vi "Select ch str (SubVI).vi"(10 "字符串":string, 11 "config":T1={"initialize"=enum."SR830", "6221"={"6221 Resource"="GPIB0::24::INSTR", "Delta status"=FALSE, "电流|RMS(A)"=0.0}, "SR830+6221"={"source"=0, "Current(A)"=0.0, "阻抗(Ohm)"=0.0, "SR830 1"=FALSE, "SR830 2"=FALSE, "SR830 3"=FALSE, "SR830 4"=FALSE, "VISA 1"="", "VISA 2"="", "VISA 3"="", "VISA 4"="", "Reserve 1"=0, "Reserve 2"=-1, "Reserve 3"=-1, "Reserve 4"=-1, "Sensitivity 1"=-1, "Sensitivity 2"=0, "Sensitivity 3"=-1, "Sensitivity 4"=-1, "量程入 1"=0, "量程入 2"=0, "量程入 3"=0, "量程入 4"=0}, "2400"={"2400"=FALSE, "VISA"="", "Output Level (0)"=1e-05, "Compliance  Level (0.1)"=10.0, "ch"=[]}, "ch"={"ch"=[], "current"=[], "change?"=[], "holding current\nwhen change ch?"=FALSE, "current offset"=[]}, "Instrument"={"limit"={"Field limit"=0.0, "Field rate limit"=0.0, "Temp limit"=0.0, "Temp low limit"=0.0, "Temp rate limit "=0.0}, "genarl"={"行数"=refnum, "编辑列表框？"=refnum, "列表框"=refnum, "camg 振荡状态"=refnum, "Aborting"=refnum, "数据文件"=refnum, "warning"=refnum, "vi路径"="", "Instrument Type"=enum."PPMS-Rotate"}, "cmag"={"TM620"="TCPIP0::192.168.1.5::4266::SOCKET", "M24C Resource"="GPIB0::24::INSTR", "4G supply"="", "Temp Status 24C"=refnum, "Temp"=refnum, "9T信号"=refnum, "4g supply status"=refnum, "in-plane"="", "out-plane"="", "in-plane signal"=FALSE, "out-plane signal"=FALSE, "in plane 信号"=refnum, "pzt volt"=refnum, "camg Rate"=refnum}, "lengtou2"={"750 visa"="", "750 rotate"="", "semaphore 340"=refnum, "semaphore 750"=refnum, "750 field status"=refnum, "Input (0:A) 340"=0, "340 Resource"="GPIB0::14::INSTR", "340 Status"=refnum, "Input (0:B) 340"=1, "Loop (0: 1)"=0, "Loop (1: 1)"=0, "TCP master instance"=refnum}, "lengtou"={"TCP master instance"=refnum, "335 Status"=refnum, "335 Resource "="GPIB0::24::INSTR", "Input (0:A) 335"=0, "Input (0:B) 335"=1, "Heater Output (1:1) 335"=1, "semaphore 335"=refnum}, "325 for test"={"quantum design"=refnum, "semaphore 325"=refnum, "325 Resource "="GPIB0::13::INSTR", "Input (0:A) 325"=0, "Heater Output (1:1) 325"=1, "325 Status"=refnum}}, "2614B"={"2614B chA"=FALSE, "2614B chB"=FALSE, "VISA"=""}, "33522b"={"33522b resource name"="", "零电压"=0.0, "最大电压"=148.0, "间隔"=4.0, "最小电压"=-48.0, "loop"=0.0, "压电陶瓷电压(Vpp)"=0.0}, "gating type"=enum."2614(daul)", "层数"=0, "行数"=0, "是否处理"=[], "current 2"=[]} {"Instrument"."325 for test"."Heater Output (1:1) 325" items=["1"=1, "2"=2]; "Instrument"."325 for test"."Input (0:A) 325" items=["A", "B"]; "Instrument"."lengtou"."Heater Output (1:1) 335" items=["1"=1, "2"=2]; "Instrument"."lengtou"."Input (0:B) 335" items=["A", "B"]; "Instrument"."lengtou"."Input (0:A) 335" items=["A", "B"]; "Instrument"."lengtou2"."Loop (1: 1)" items=["1", "2"]; "Instrument"."lengtou2"."Loop (0: 1)" items=["1", "2"]; "Instrument"."lengtou2"."Input (0:B) 340" items=["A", "B", "C", "D"]; "Instrument"."lengtou2"."Input (0:A) 340" items=["A", "B", "C", "D"]; "SR830+6221"."Sensitivity 4" items=["Auto Gain"=-1, "2 nV/fA"=0, "5 nV/fA"=1, "10 nV/fA"=2, "20 nV/fA"=3, "50 nV/fA"=4, "100 nV/fA"=5, "200 nV/fA"=6, "500 nV/fA"=7, "1 uV/pA"=8, "2 uV/pA"=9, "5 uV/pA"=10, "10 uV/pA"=11, "20 uV/pA"=12, "50 uV/pA"=13, "100 uV/pA"=14, "200 uV/pA"=15, "500 uV/pA"=16, "1 mV/nA"=17, "2 mV/nA"=18, "5 mV/nA"=19, "10 mV/nA"=20, "20 mV/nA"=21, "50 mV/nA"=22, "100 mV/nA"=23, "200 mV/nA"=24, "500 mV/mA"=25, "1 V/uA"=26]; "SR830+6221"."Sensitivity 3" items=["Auto Gain"=-1, "2 nV/fA"=0, "5 nV/fA"=1, "10 nV/fA"=2, "20 nV/fA"=3, "50 nV/fA"=4, "100 nV/fA"=5, "200 nV/fA"=6, "500 nV/fA"=7, "1 uV/pA"=8, "2 uV/pA"=9, "5 uV/pA"=10, "10 uV/pA"=11, "20 uV/pA"=12, "50 uV/pA"=13, "100 uV/pA"=14, "200 uV/pA"=15, "500 uV/pA"=16, "1 mV/nA"=17, "2 mV/nA"=18, "5 mV/nA"=19, "10 mV/nA"=20, "20 mV/nA"=21, "50 mV/nA"=22, "100 mV/nA"=23, "200 mV/nA"=24, "500 mV/mA"=25, "1 V/uA"=26]; "SR830+6221"."Sensitivity 1" items=["Auto Gain"=-1, "2 nV/fA"=0, "5 nV/fA"=1, "10 nV/fA"=2, "20 nV/fA"=3, "50 nV/fA"=4, "100 nV/fA"=5, "200 nV/fA"=6, "500 nV/fA"=7, "1 uV/pA"=8, "2 uV/pA"=9, "5 uV/pA"=10, "10 uV/pA"=11, "20 uV/pA"=12, "50 uV/pA"=13, "100 uV/pA"=14, "200 uV/pA"=15, "500 uV/pA"=16, "1 mV/nA"=17, "2 mV/nA"=18, "5 mV/nA"=19, "10 mV/nA"=20, "20 mV/nA"=21, "50 mV/nA"=22, "100 mV/nA"=23, "200 mV/nA"=24, "500 mV/mA"=25, "1 V/uA"=26]; "SR830+6221"."Sensitivity 2" items=["Auto Gain"=-1, "2 nV/fA"=0, "5 nV/fA"=1, "10 nV/fA"=2, "20 nV/fA"=3, "50 nV/fA"=4, "100 nV/fA"=5, "200 nV/fA"=6, "500 nV/fA"=7, "1 uV/pA"=8, "2 uV/pA"=9, "5 uV/pA"=10, "10 uV/pA"=11, "20 uV/pA"=12, "50 uV/pA"=13, "100 uV/pA"=14, "200 uV/pA"=15, "500 uV/pA"=16, "1 mV/nA"=17, "2 mV/nA"=18, "5 mV/nA"=19, "10 mV/nA"=20, "20 mV/nA"=21, "50 mV/nA"=22, "100 mV/nA"=23, "200 mV/nA"=24, "500 mV/mA"=25, "1 V/uA"=26]; "SR830+6221"."Reserve 4" items=["Auto Gain"=-1, "2 nV/fA"=0, "5 nV/fA"=1, "10 nV/fA"=2, "20 nV/fA"=3, "50 nV/fA"=4, "100 nV/fA"=5, "200 nV/fA"=6, "500 nV/fA"=7, "1 uV/pA"=8, "2 uV/pA"=9, "5 uV/pA"=10, "10 uV/pA"=11, "20 uV/pA"=12, "50 uV/pA"=13, "100 uV/pA"=14, "200 uV/pA"=15, "500 uV/pA"=16, "1 mV/nA"=17, "2 mV/nA"=18, "5 mV/nA"=19, "10 mV/nA"=20, "20 mV/nA"=21, "50 mV/nA"=22, "100 mV/nA"=23, "200 mV/nA"=24, "500 mV/mA"=25, "1 V/uA"=26]; "SR830+6221"."Reserve 3" items=["Auto Reserve"=-1, "High Reserve"=0, "Normal"=1, "Low Noise"=2]; "SR830+6221"."Reserve 2" items=["Auto Reserve"=-1, "High Reserve"=0, "Normal"=1, "Low Noise"=2]; "SR830+6221"."Reserve 1" items=["Auto Reserve"=-1, "High Reserve"=0, "Normal"=1, "Low Noise"=2]; "SR830+6221"."source" items=["SR830 1", "SR830 2", "SR830 3", "SR830 4"]}) -> (3 "config out":T1={"initialize"=enum."SR830", "6221"={"6221 Resource"="GPIB0::24::INSTR", "Delta status"=FALSE, "电流|RMS(A)"=0.0}, "SR830+6221"={"source"=0, "Current(A)"=0.0, "阻抗(Ohm)"=0.0, "SR830 1"=FALSE, "SR830 2"=FALSE, "SR830 3"=FALSE, "SR830 4"=FALSE, "VISA 1"="", "VISA 2"="", "VISA 3"="", "VISA 4"="", "Reserve 1"=0, "Reserve 2"=-1, "Reserve 3"=-1, "Reserve 4"=-1, "Sensitivity 1"=-1, "Sensitivity 2"=0, "Sensitivity 3"=-1, "Sensitivity 4"=-1, "量程入 1"=0, "量程入 2"=0, "量程入 3"=0, "量程入 4"=0}, "2400"={"2400"=FALSE, "VISA"="", "Output Level (0)"=1e-05, "Compliance  Level (0.1)"=10.0, "ch"=[]}, "ch"={"ch"=[], "current"=[], "change?"=[], "holding current\nwhen change ch?"=FALSE, "current offset"=[]}, "Instrument"={"limit"={"Field limit"=0.0, "Field rate limit"=0.0, "Temp limit"=0.0, "Temp low limit"=0.0, "Temp rate limit "=0.0}, "genarl"={"行数"=refnum, "编辑列表框？"=refnum, "列表框"=refnum, "camg 振荡状态"=refnum, "Aborting"=refnum, "数据文件"=refnum, "warning"=refnum, "vi路径"="", "Instrument Type"=enum."PPMS-Rotate"}, "cmag"={"TM620"="TCPIP0::192.168.1.5::4266::SOCKET", "M24C Resource"="GPIB0::24::INSTR", "4G supply"="", "Temp Status 24C"=refnum, "Temp"=refnum, "9T信号"=refnum, "4g supply status"=refnum, "in-plane"="", "out-plane"="", "in-plane signal"=FALSE, "out-plane signal"=FALSE, "in plane 信号"=refnum, "pzt volt"=refnum, "camg Rate"=refnum}, "lengtou2"={"750 visa"="", "750 rotate"="", "semaphore 340"=refnum, "semaphore 750"=refnum, "750 field status"=refnum, "Input (0:A) 340"=0, "340 Resource"="GPIB0::14::INSTR", "340 Status"=refnum, "Input (0:B) 340"=1, "Loop (0: 1)"=0, "Loop (1: 1)"=0, "TCP master instance"=refnum}, "lengtou"={"TCP master instance"=refnum, "335 Status"=refnum, "335 Resource "="GPIB0::24::INSTR", "Input (0:A) 335"=0, "Input (0:B) 335"=1, "Heater Output (1:1) 335"=1, "semaphore 335"=refnum}, "325 for test"={"quantum design"=refnum, "semaphore 325"=refnum, "325 Resource "="GPIB0::13::INSTR", "Input (0:A) 325"=0, "Heater Output (1:1) 325"=1, "325 Status"=refnum}}, "2614B"={"2614B chA"=FALSE, "2614B chB"=FALSE, "VISA"=""}, "33522b"={"33522b resource name"="", "零电压"=0.0, "最大电压"=148.0, "间隔"=4.0, "最小电压"=-48.0, "loop"=0.0, "压电陶瓷电压(Vpp)"=0.0}, "gating type"=enum."2614(daul)", "层数"=0, "行数"=0, "是否处理"=[], "current 2"=[]} {"Instrument"."325 for test"."Heater Output (1:1) 325" items=["1"=1, "2"=2]; "Instrument"."325 for test"."Input (0:A) 325" items=["A", "B"]; "Instrument"."lengtou"."Heater Output (1:1) 335" items=["1"=1, "2"=2]; "Instrument"."lengtou"."Input (0:B) 335" items=["A", "B"]; "Instrument"."lengtou"."Input (0:A) 335" items=["A", "B"]; "Instrument"."lengtou2"."Loop (1: 1)" items=["1", "2"]; "Instrument"."lengtou2"."Loop (0: 1)" items=["1", "2"]; "Instrument"."lengtou2"."Input (0:B) 340" items=["A", "B", "C", "D"]; "Instrument"."lengtou2"."Input (0:A) 340" items=["A", "B", "C", "D"]; "SR830+6221"."Sensitivity 4" items=["Auto Gain"=-1, "2 nV/fA"=0, "5 nV/fA"=1, "10 nV/fA"=2, "20 nV/fA"=3, "50 nV/fA"=4, "100 nV/fA"=5, "200 nV/fA"=6, "500 nV/fA"=7, "1 uV/pA"=8, "2 uV/pA"=9, "5 uV/pA"=10, "10 uV/pA"=11, "20 uV/pA"=12, "50 uV/pA"=13, "100 uV/pA"=14, "200 uV/pA"=15, "500 uV/pA"=16, "1 mV/nA"=17, "2 mV/nA"=18, "5 mV/nA"=19, "10 mV/nA"=20, "20 mV/nA"=21, "50 mV/nA"=22, "100 mV/nA"=23, "200 mV/nA"=24, "500 mV/mA"=25, "1 V/uA"=26]; "SR830+6221"."Sensitivity 3" items=["Auto Gain"=-1, "2 nV/fA"=0, "5 nV/fA"=1, "10 nV/fA"=2, "20 nV/fA"=3, "50 nV/fA"=4, "100 nV/fA"=5, "200 nV/fA"=6, "500 nV/fA"=7, "1 uV/pA"=8, "2 uV/pA"=9, "5 uV/pA"=10, "10 uV/pA"=11, "20 uV/pA"=12, "50 uV/pA"=13, "100 uV/pA"=14, "200 uV/pA"=15, "500 uV/pA"=16, "1 mV/nA"=17, "2 mV/nA"=18, "5 mV/nA"=19, "10 mV/nA"=20, "20 mV/nA"=21, "50 mV/nA"=22, "100 mV/nA"=23, "200 mV/nA"=24, "500 mV/mA"=25, "1 V/uA"=26]; "SR830+6221"."Sensitivity 1" items=["Auto Gain"=-1, "2 nV/fA"=0, "5 nV/fA"=1, "10 nV/fA"=2, "20 nV/fA"=3, "50 nV/fA"=4, "100 nV/fA"=5, "200 nV/fA"=6, "500 nV/fA"=7, "1 uV/pA"=8, "2 uV/pA"=9, "5 uV/pA"=10, "10 uV/pA"=11, "20 uV/pA"=12, "50 uV/pA"=13, "100 uV/pA"=14, "200 uV/pA"=15, "500 uV/pA"=16, "1 mV/nA"=17, "2 mV/nA"=18, "5 mV/nA"=19, "10 mV/nA"=20, "20 mV/nA"=21, "50 mV/nA"=22, "100 mV/nA"=23, "200 mV/nA"=24, "500 mV/mA"=25, "1 V/uA"=26]; "SR830+6221"."Sensitivity 2" items=["Auto Gain"=-1, "2 nV/fA"=0, "5 nV/fA"=1, "10 nV/fA"=2, "20 nV/fA"=3, "50 nV/fA"=4, "100 nV/fA"=5, "200 nV/fA"=6, "500 nV/fA"=7, "1 uV/pA"=8, "2 uV/pA"=9, "5 uV/pA"=10, "10 uV/pA"=11, "20 uV/pA"=12, "50 uV/pA"=13, "100 uV/pA"=14, "200 uV/pA"=15, "500 uV/pA"=16, "1 mV/nA"=17, "2 mV/nA"=18, "5 mV/nA"=19, "10 mV/nA"=20, "20 mV/nA"=21, "50 mV/nA"=22, "100 mV/nA"=23, "200 mV/nA"=24, "500 mV/mA"=25, "1 V/uA"=26]; "SR830+6221"."Reserve 4" items=["Auto Gain"=-1, "2 nV/fA"=0, "5 nV/fA"=1, "10 nV/fA"=2, "20 nV/fA"=3, "50 nV/fA"=4, "100 nV/fA"=5, "200 nV/fA"=6, "500 nV/fA"=7, "1 uV/pA"=8, "2 uV/pA"=9, "5 uV/pA"=10, "10 uV/pA"=11, "20 uV/pA"=12, "50 uV/pA"=13, "100 uV/pA"=14, "200 uV/pA"=15, "500 uV/pA"=16, "1 mV/nA"=17, "2 mV/nA"=18, "5 mV/nA"=19, "10 mV/nA"=20, "20 mV/nA"=21, "50 mV/nA"=22, "100 mV/nA"=23, "200 mV/nA"=24, "500 mV/mA"=25, "1 V/uA"=26]; "SR830+6221"."Reserve 3" items=["Auto Reserve"=-1, "High Reserve"=0, "Normal"=1, "Low Noise"=2]; "SR830+6221"."Reserve 2" items=["Auto Reserve"=-1, "High Reserve"=0, "Normal"=1, "Low Noise"=2]; "SR830+6221"."Reserve 1" items=["Auto Reserve"=-1, "High Reserve"=0, "Normal"=1, "Low Noise"=2]; "SR830+6221"."source" items=["SR830 1", "SR830 2", "SR830 3", "SR830 4"]})   [LabVIEW 2019, in "Take Seq.lvlib"]
uses:
  Take Seq.lvlib
  ctl/config.ctl
  <vilib>/NI/Modbus Library/API/Master/Modbus Master.lvclass
  ctl/initialize.ctl
  ctl/Instrument.ctl
  ctl/limit.ctl
  ctl/warning.ctl
  ctl/Instrument Type.ctl
  ctl/335 state.ctl
  ctl/9T mag field stauts.ctl
  C:/Users/fuyang/Desktop/postdoctor/labview/labview-measure/lib/QDInstrument.dll
  lib/QDInstrument.dll
  ctl/Gating type.ctl
  SubVI.lvlib
  lib/Keithley 622x/Keithley 622x.lvlib
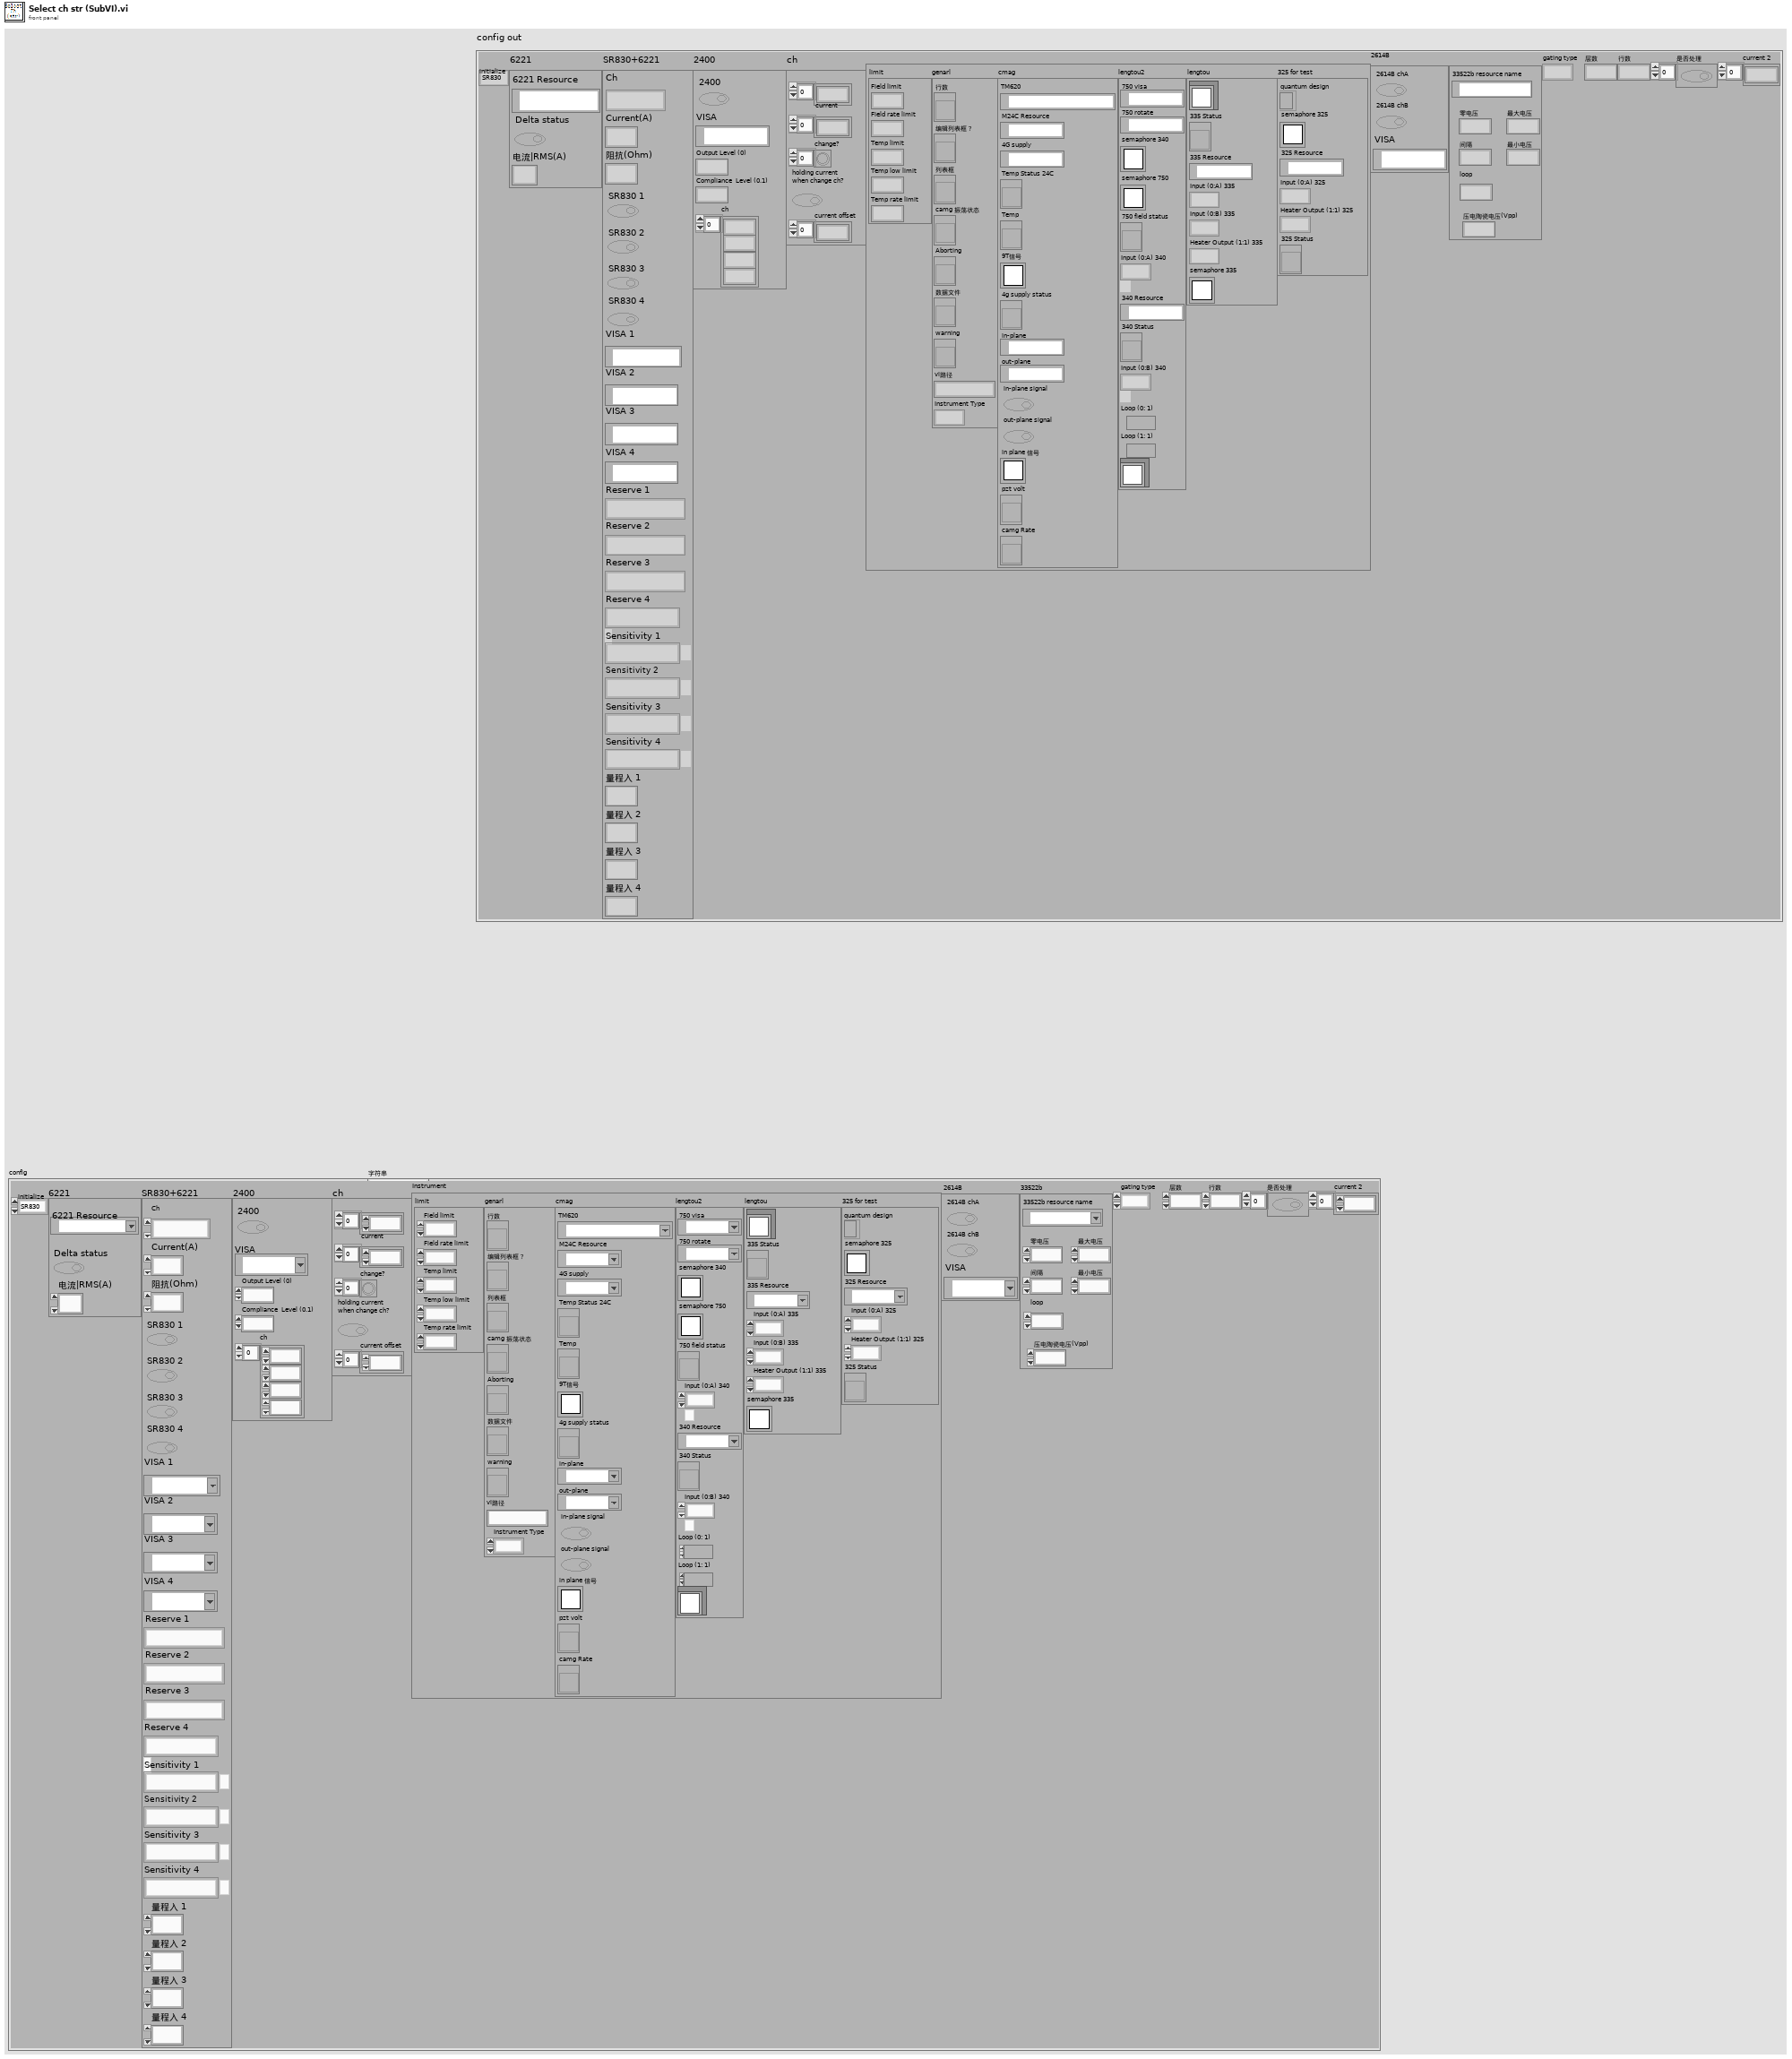
[diagram p1: front panel]
types:
  T1 = typedef "config.ctl" = cluster{"initialize":T2, "6221":cluster{"6221 Resource":refnum<visa-resource-name>, "Delta status":bool, "电流|RMS(A)":dbl}, "SR830+6221":cluster{"source":u16, "Current(A)":dbl, "阻抗(Ohm)":dbl, "SR830 1":bool, "SR830 2":bool, "SR830 3":bool, "SR830 4":bool, "VISA 1":refnum<visa-resource-name>, "VISA 2":refnum<visa-resource-name>, "VISA 3":refnum<visa-resource-name>, "VISA 4":refnum<visa-resource-name>, "Reserve 1":i16, "Reserve 2":i16, "Reserve 3":i16, "Reserve 4":i16, "Sensitivity 1":i16, "Sensitivity 2":i16, "Sensitivity 3":i16, "Sensitivity 4":i16, "量程入 1":i32, "量程入 2":i32, "量程入 3":i32, "量程入 4":i32}, "2400":cluster{"2400":bool, "VISA":refnum<visa-resource-name>, "Output Level (0)":dbl, "Compliance  Level (0.1)":dbl, "ch":i32[]}, "ch":cluster{"ch":i32[], "current":dbl[], "change?":bool[], "holding current\nwhen change ch?":bool, "current offset":dbl[]}, "Instrument":T3, "2614B":cluster{"2614B chA":bool, "2614B chB":bool, "VISA":refnum<visa-resource-name>}, "33522b":cluster{"33522b resource name":refnum<visa-resource-name>, "零电压":dbl, "最大电压":dbl, "间隔":dbl, "最小电压":dbl, "loop":dbl, "压电陶瓷电压(Vpp)":dbl}, "gating type":T7, "层数":i32, "行数":i32, "是否处理":bool[], "current 2":dbl[]}
  T2 = typedef "initialize.ctl" = enum16{"SR830", "keithley6221-SR830", "Delta", "Delta-tunnelling", "keithley6221-2182-DC", "PZT", "4200"}
  T3 = typedef "Instrument.ctl" = cluster{"limit":T4, "genarl":cluster{"行数":refnum<vi>, "编辑列表框？":refnum<vi>, "列表框":refnum<vi>, "camg 振荡状态":refnum<vi>, "Aborting":refnum<vi>, "数据文件":refnum<vi>, "warning":refnum<vi>, "vi路径":string, "Instrument Type":T5}, "cmag":cluster{"TM620":refnum<visa-resource-name>, "M24C Resource":refnum<visa-resource-name>, "4G supply":refnum<visa-resource-name>, "Temp Status 24C":refnum<vi>, "Temp":refnum<vi>, "9T信号":T6, "4g supply status":refnum<vi>, "in-plane":refnum<visa-resource-name>, "out-plane":refnum<visa-resource-name>, "in-plane signal":bool, "out-plane signal":bool, "in plane 信号":T6, "pzt volt":refnum<vi>, "camg Rate":refnum<vi>}, "lengtou2":cluster{"750 visa":refnum<visa-resource-name>, "750 rotate":refnum<visa-resource-name>, "semaphore 340":T6, "semaphore 750":T6, "750 field status":refnum<vi>, "Input (0:A) 340":u16, "340 Resource":refnum<visa-resource-name>, "340 Status":refnum<vi>, "Input (0:B) 340":u16, "Loop (0: 1)":u16, "Loop (1: 1)":u16, "TCP master instance":refnum<class "Modbus Master.lvclass">}, "lengtou":cluster{"TCP master instance":refnum<class "Modbus Master.lvclass">, "335 Status":refnum<vi>, "335 Resource ":refnum<visa-resource-name>, "Input (0:A) 335":u16, "Input (0:B) 335":u16, "Heater Output (1:1) 335":u16, "semaphore 335":T6}, "325 for test":cluster{"quantum design":refnum<k24>, "semaphore 325":T6, "325 Resource ":refnum<visa-resource-name>, "Input (0:A) 325":u16, "Heater Output (1:1) 325":u16, "325 Status":refnum<vi>}}
  T4 = typedef "limit.ctl" = cluster{"Field limit":dbl, "Field rate limit":dbl, "Temp limit":dbl, "Temp low limit":dbl, "Temp rate limit ":dbl}
  T5 = typedef "Instrument Type.ctl" = enum16{"PPMS", "VersaLab", "DynaCool", "SVSM", "PPMS-Rotate", "Lakeshore335", "lengtou2", "9T mag old", "9T cmag", "9T cmag DAC", "9T cmag rotate", "test"}
  T6 = typedef "Semaphore RefNum" = refnum<k1>
  T7 = typedef "Gating type.ctl" = enum32{"null", "2614(daul)", "2400", "6517B"}
  T8 = cluster{"ch":i32[], "current":dbl[], "change?":bool[], "holding current\nwhen change ch?":bool, "current offset":dbl[]}
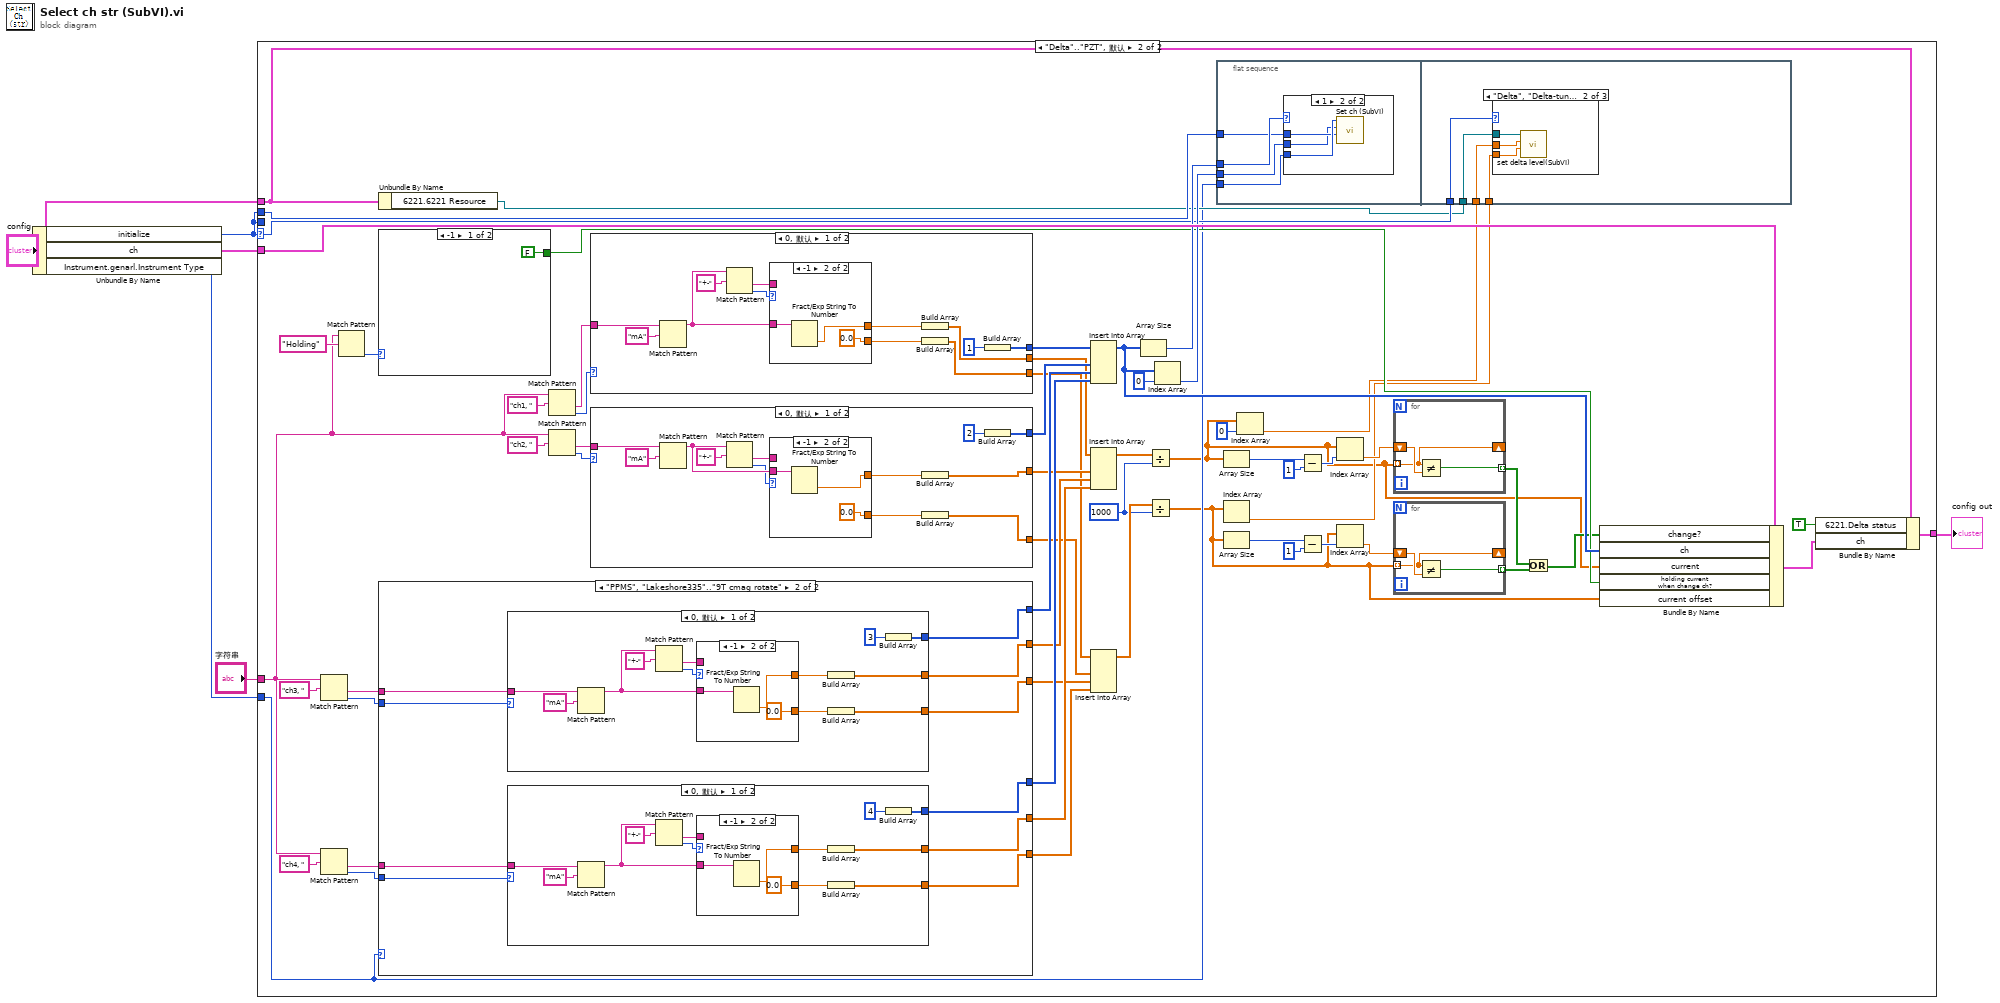
[diagram p0: block diagram]
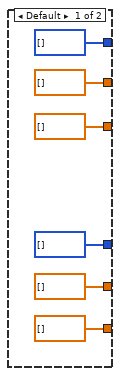
[diagram p3: hidden frame]
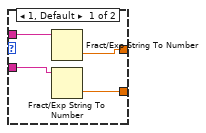
[diagram p4: hidden frame]
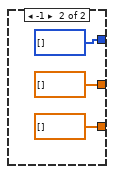
[diagram p5: hidden frame]
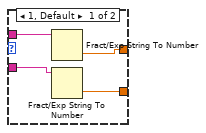
[diagram p6: hidden frame]
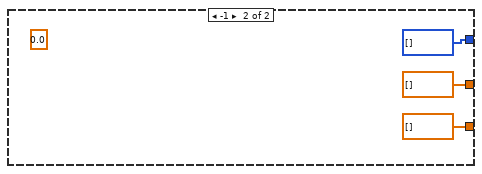
[diagram p7: hidden frame]
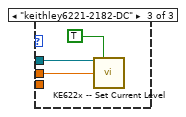
[diagram p10: hidden frame]
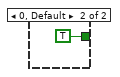
[diagram p11: hidden frame]
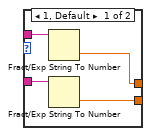
[diagram p12: hidden frame]
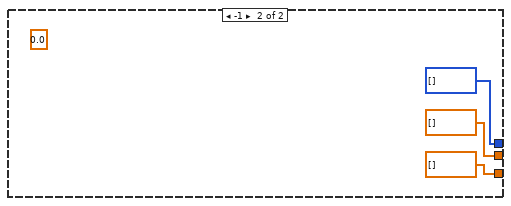
[diagram p13: hidden frame]
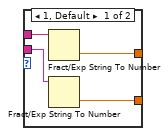
[diagram p14: hidden frame]
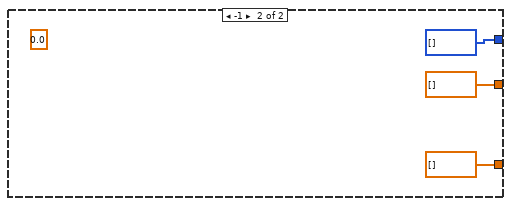
[diagram p15: hidden frame]
diagram:
  n1 = Unbundle By Name("config") -> ("initialize"=w2:T2, "ch"=w3:T8, "Instrument.genarl.Instrument Type"=w1:T5)
  n2 = case shown="\"Delta\"..\"PZT\", 默认" w2 {
    selector: w2 -> [_ w28]
    tunnel: "字符串" -> [_ w30]
    tunnel: w2 -> [_ _]
    tunnel: "config" -> [w7 w52]
    tunnel: [w7 w50] -> w4
    tunnel: w3 -> [_ w61]
    tunnel: w2 -> [_ w46]
    tunnel: w1 -> [_ w25]
    frame "SR830", "keithley6221-SR830" {
    }
    frame "Delta".."PZT", Default {
      w9 = 1000
      n3 = Match Pattern(string=w30, regular expression="ch3, " ("正则表达式")) -> (after substring=w58:string, offset past match=w55:i32)  [unwired: 1 in, 2 out]
      n4 = Match Pattern(string=w30, regular expression="ch4, " ("正则表达式")) -> (after substring=w57:string, offset past match=w56:i32)  [unwired: 1 in, 2 out]
      n5 = Match Pattern(string=w30, regular expression="Holding" ("正则表达式")) -> (offset past match=w31:i32)  [unwired: 1 in, 3 out]
      n6 = Unbundle By Name(w52) -> ("6221.6221 Resource"=w27:refnum<visa-resource-name>)
      n7 = case shown="-1" w31 {
        tunnel: [FALSE TRUE] -> w29
        frame -1 {
        }
        frame 0, Default {
        }
      }
      n8 = case shown="\"PPMS\", \"Lakeshore335\"..\"9T cmag rotate\"" w25 {
        tunnel: w58 -> [_ w86]
        tunnel: w57 -> [_ w85]
        tunnel: w56 -> [_ w84]
        tunnel: w55 -> [_ w83]
        tunnel: [i32[] [] w82] -> w42
        tunnel: [i32[] [] w81] -> w41
        tunnel: [dbl[] [] w80] -> w37
        tunnel: [dbl[] [] w79] -> w36
        tunnel: [dbl[] [] w78] -> w22
        tunnel: [dbl[] [] w77] -> w21
        frame Default {
        }
        frame "PPMS", "Lakeshore335".."9T cmag rotate" {
          n9 = case shown="0, 默认" w83 {
            tunnel: w86 -> [w120 _]
            tunnel: [w116 dbl[] []] -> w80
            tunnel: [w117 i32[] []] -> w82
            tunnel: [w114 dbl[] []] -> w78
            frame 0, Default {
              n10 = Match Pattern(string=w120, regular expression="mA" ("正则表达式")) -> (before substring=w112:string)  [unwired: 1 in, 3 out]
              n11 = Match Pattern(string=w112, regular expression="+-" ("正则表达式")) -> (after substring=w113:string, offset past match=w111:i32)  [unwired: 1 in, 2 out]
              n12 = case shown="-1" w111 {
                tunnel: w113 -> [w124 _]
                tunnel: w112 -> [w123 w127]
                tunnel: [w122 0.0] -> w109
                tunnel: [w121 w126] -> w110
                frame 1, Default {
                  n13 = Fract/Exp String To Number(string=w124) -> (number=w121:dbl)  [unwired: 3 in, 1 out]
                  n14 = Fract/Exp String To Number(string=w123) -> (number=w122:dbl)  [unwired: 3 in, 1 out]
                }
                frame -1 {
                  n15 = Fract/Exp String To Number(string=w127) -> (number=w126:dbl)  [unwired: 3 in, 1 out]
                }
              }
              n16 = Build Array(w110) -> (w116:dbl[])
              n17 = Build Array(w109) -> (w114:dbl[])
              n18 = Build Array(3) -> (w117:i32[])
            }
            frame -1 {
              (unwired) 0.0
            }
          }
          n19 = case shown="0, 默认" w84 {
            tunnel: w85 -> [w98 _]
            tunnel: [w94 dbl[] []] -> w79
            tunnel: [w95 i32[] []] -> w81
            tunnel: [w92 dbl[] []] -> w77
            frame 0, Default {
              n20 = Match Pattern(string=w98, regular expression="mA" ("正则表达式")) -> (before substring=w90:string)  [unwired: 1 in, 3 out]
              n21 = Match Pattern(string=w90, regular expression="+-" ("正则表达式")) -> (after substring=w91:string, offset past match=w87:i32)  [unwired: 1 in, 2 out]
              n22 = case shown="-1" w87 {
                tunnel: w91 -> [w102 _]
                tunnel: w90 -> [w101 w105]
                tunnel: [w100 0.0] -> w89
                tunnel: [w99 w104] -> w88
                frame 1, Default {
                  n23 = Fract/Exp String To Number(string=w102) -> (number=w99:dbl)  [unwired: 3 in, 1 out]
                  n24 = Fract/Exp String To Number(string=w101) -> (number=w100:dbl)  [unwired: 3 in, 1 out]
                }
                frame -1 {
                  n25 = Fract/Exp String To Number(string=w105) -> (number=w104:dbl)  [unwired: 3 in, 1 out]
                }
              }
              n26 = Build Array(w88) -> (w94:dbl[])
              n27 = Build Array(w89) -> (w92:dbl[])
              n28 = Build Array(4) -> (w95:i32[])
            }
            frame -1 {
            }
          }
        }
      }
      n29 = Match Pattern(string=w30, regular expression="ch1, " ("正则表达式")) -> (after substring=w59:string, offset past match=w60:i32)  [unwired: 1 in, 2 out]
      n30 = Match Pattern(string=w30, regular expression="ch2, " ("正则表达式")) -> (after substring=w62:string, offset past match=w63:i32)  [unwired: 1 in, 2 out]
      n31 = case shown="0, 默认" w60 {
        tunnel: w59 -> [w164 _]
        tunnel: [w160 dbl[] []] -> w39
        tunnel: [w161 i32[] []] -> w44
        tunnel: [w158 dbl[] []] -> w24
        frame 0, Default {
          n32 = Match Pattern(string=w164, regular expression="mA" ("正则表达式")) -> (before substring=w157:string)  [unwired: 1 in, 3 out]
          n33 = Match Pattern(string=w157, regular expression="+-" ("正则表达式")) -> (after substring=w156:string, offset past match=w153:i32)  [unwired: 1 in, 2 out]
          n34 = case shown="-1" w153 {
            tunnel: w156 -> [w168 _]
            tunnel: w157 -> [w167 w171]
            tunnel: [w166 0.0] -> w154
            tunnel: [w165 w170] -> w155
            frame 1, Default {
              n35 = Fract/Exp String To Number(string=w168) -> (number=w165:dbl)  [unwired: 3 in, 1 out]
              n36 = Fract/Exp String To Number(string=w167) -> (number=w166:dbl)  [unwired: 3 in, 1 out]
            }
            frame -1 {
              n37 = Fract/Exp String To Number(string=w171) -> (number=w170:dbl)  [unwired: 3 in, 1 out]
            }
          }
          n38 = Build Array(w155) -> (w160:dbl[])
          n39 = Build Array(w154) -> (w158:dbl[])
          n40 = Build Array(1) -> (w161:i32[])
        }
        frame -1 {
          (unwired) 0.0
        }
      }
      n41 = case shown="0, 默认" w63 {
        tunnel: w62 -> [w186 _]
        tunnel: [w182 dbl[] []] -> w38
        tunnel: [w183 i32[] []] -> w43
        tunnel: [w180 dbl[] []] -> w23
        frame 0, Default {
          n42 = Match Pattern(string=w186, regular expression="mA" ("正则表达式")) -> (before substring=w178:string)  [unwired: 1 in, 3 out]
          n43 = Match Pattern(string=w178, regular expression="+-" ("正则表达式")) -> (after substring=w179:string, offset past match=w175:i32)  [unwired: 1 in, 2 out]
          n44 = case shown="-1" w175 {
            tunnel: w179 -> [w190 _]
            tunnel: w178 -> [w189 w193]
            tunnel: [w188 0.0] -> w176
            tunnel: [w187 w192] -> w177
            frame 1, Default {
              n45 = Fract/Exp String To Number(string=w190) -> (number=w187:dbl)  [unwired: 3 in, 1 out]
              n46 = Fract/Exp String To Number(string=w189) -> (number=w188:dbl)  [unwired: 3 in, 1 out]
            }
            frame -1 {
              n47 = Fract/Exp String To Number(string=w193) -> (number=w192:dbl)  [unwired: 3 in, 1 out]
            }
          }
          n48 = Build Array(w177) -> (w182:dbl[])
          n49 = Build Array(w176) -> (w180:dbl[])
          n50 = Build Array(2) -> (w183:i32[])
        }
        frame -1 {
          (unwired) 0.0
        }
      }
      n51 = Insert Into Array(array=w44, new element #1=w43, new element #2=w42, new element #3=w41) -> (w40:i32[])  [unwired: 1 in]
      n52 = Insert Into Array(array=w39, new element #1=w38, new element #2=w37, new element #3=w36) -> (w10:dbl[])  [unwired: 1 in]
      n53 = Insert Into Array(array=w24, new element #1=w23, new element #2=w22, new element #3=w21) -> (w12:dbl[])  [unwired: 1 in]
      n54 = Array Size(array=w40) -> (size(s)=w48:i32)
      n55 = Divide(x=w10, y=w9) -> (x/y=w8:dbl[])
      n56 = Divide(x=w12, y=w9) -> (x/y=w11:dbl[])
      n57 = Index Array(array=w40, index=0 ("索引")) -> (element=w45:i32)
      n58 = flat-sequence {
        tunnel: w48 -> [w134]
        tunnel: w25 -> [w133]
        tunnel: w46 -> [w132]
        tunnel: w45 -> [w131]
        tunnel: w28 -> [w141]
        tunnel: w27 -> [w140]
        tunnel: w26 -> [w139]
        tunnel: w13 -> [w138]
        frame #0 {
          n59 = case shown="1" w134 {
            tunnel: w133 -> [_ w137]
            tunnel: w132 -> [_ w136]
            tunnel: w131 -> [_ w135]
            frame 0, Default {
            }
            frame 1 {
              n60 = call "Set ch (SubVI).vi"("initialize"=w136, "数值"=w135, "Instrument Type"=w137) -> ()  [unwired: 9 in]
            }
          }
        }
        frame #1 {
          n61 = case shown="\"Delta\", \"Delta-tunnelling\", \"PZT\", 默认" w141 {
            tunnel: w140 -> [_ w144 w146]
            tunnel: w139 -> [_ w143 w147]
            tunnel: w138 -> [_ w142 _]
            frame "SR830" {
            }
            frame "Delta", "Delta-tunnelling", "PZT", Default {
              n62 = call "set delta level(SubVI).vi"("current offset(A)"=w142, "电流（A）"=w143, "VISA引用句柄输入"=w144) -> ()  [unwired: 7 in, 2 out]
            }
            frame "keithley6221-2182-DC" {
              n63 = call "KE622x -- Set Current Level.vi"("Resource In"=w146, "Check For SCPI Errors? (T)"=TRUE, "Current Level (A) In"=w147) -> ()  [unwired: 10 in, 3 out]
            }
          }
        }
      }
      n64 = Array Size(array=w8) -> (size(s)=w35:i32)
      n65 = Index Array(array=w11) -> (element=w13:dbl)  [unwired: 1 in]
      n66 = Array Size(array=w11) -> (size(s)=w14:i32)
      n67 = Index Array(array=w8, index=0 ("索引")) -> (element=w26:dbl)
      n68 = Subtract(x=w35, y=1) -> (x-y=w33:i32)
      n69 = Subtract(x=w14, y=1) -> (x-y=w20:i32)
      n70 = Index Array(array=w8, index=w33) -> (element=w54:dbl)
      n71 = Index Array(array=w11, index=w20) -> (element=w18:dbl)
      n72 = for {
        tunnel: w8 -> [w150] mode=indexing
        tunnel: [w151] -> w16 mode=indexing
        shift-right: [w150] -> _
        shift-left: w54 -> [w152]
        n73 = Not Equal?(x=w150, y=w152) -> (x != y?=w151:bool)
      }
      n74 = for {
        tunnel: w11 -> [w68] mode=indexing
        tunnel: [w69] -> w17 mode=indexing
        shift-right: [w68] -> _
        shift-left: w18 -> [w70]
        n75 = Not Equal?(x=w68, y=w70) -> (x != y?=w69:bool)
      }
      n76 = Or(x=w16, y=w17) -> (x .or. y?=w15:bool[])
      n77 = Bundle By Name(cluster=w61, "change?"=w15, "ch"=w40, "current"=w8, "holding current\nwhen change ch?"=w29, "current offset"=w11) -> (w51:T8)
      n78 = Bundle By Name(cluster=w52, "6221.Delta status"=TRUE, "ch"=w51) -> (w50:T1)
    }
  }
  "config out" <- w4
